vi "LeyboldPump_word.vi"() -> ()   [LabVIEW 2015]
panel:
  in  "PZD6 - Current intermediate circuit voltage 2":string="\u0000\u0000"
  in  "Reserved x2 2":string="\u0000\u0000"
  in  "PZD4 - Current Motor Current 2":string="\u0000\u0000"
  in  "PZD3 - Current Freq Converter Temp 2":string="\u0000\u0000"
  in  "PZD2 - Current Stator Freq 2":string="\u0000\u0000"
  in  "PZD1 - Status & Control 2":string="\u0000\u0000"
  in  "PWE (Parameter Value 4Bytes) 2":string="\u0000\u0000\u0000\u0000"
  in  "IND (Parameter Index) 2":string="\u0000"
  in  "Reserved 2":string="\u0000"
  in  "PKE - 2Bytes 2":string="\u0000\u0000"
  in  "ADR 2":string="\u0000"
  in  "LGE 2":string="\u0016"
  in  "STX 2":string="\u0002"
  out "Result String":string
  out "BCC - Checksum":string
  out "PZD6 - Current intermediate circuit voltage":string
  out "Reserved x2":string
  out "PZD4 - Current Motor Current":string
  out "PZD3 - Current Freq Converter Temp":string
  out "PZD2 - Current Stator Freq":string
  out "PZD1 - Status & Control":string
  out "PWE (Parameter Value 4Bytes)":string
  out "IND (Parameter Index)":string
  out "Reserved":string
  out "PKE - 2Bytes":string
  out "ADR":string
  out "LGE":string
  out "STX":string
  in  "Input String":string
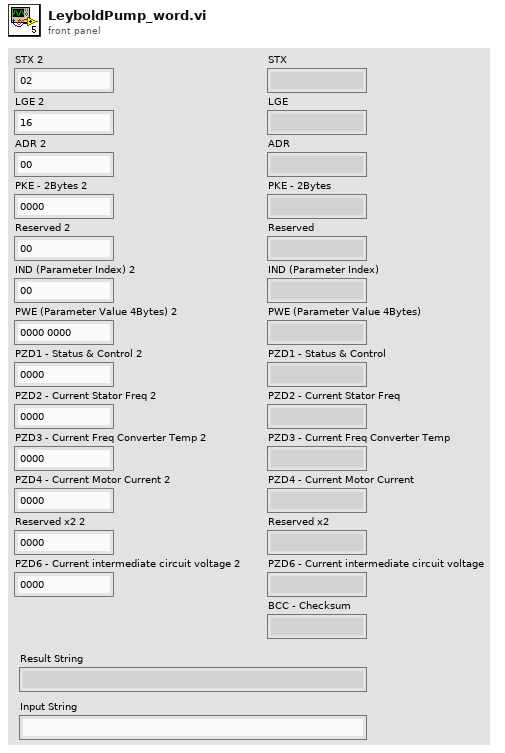
[diagram p1: front panel]
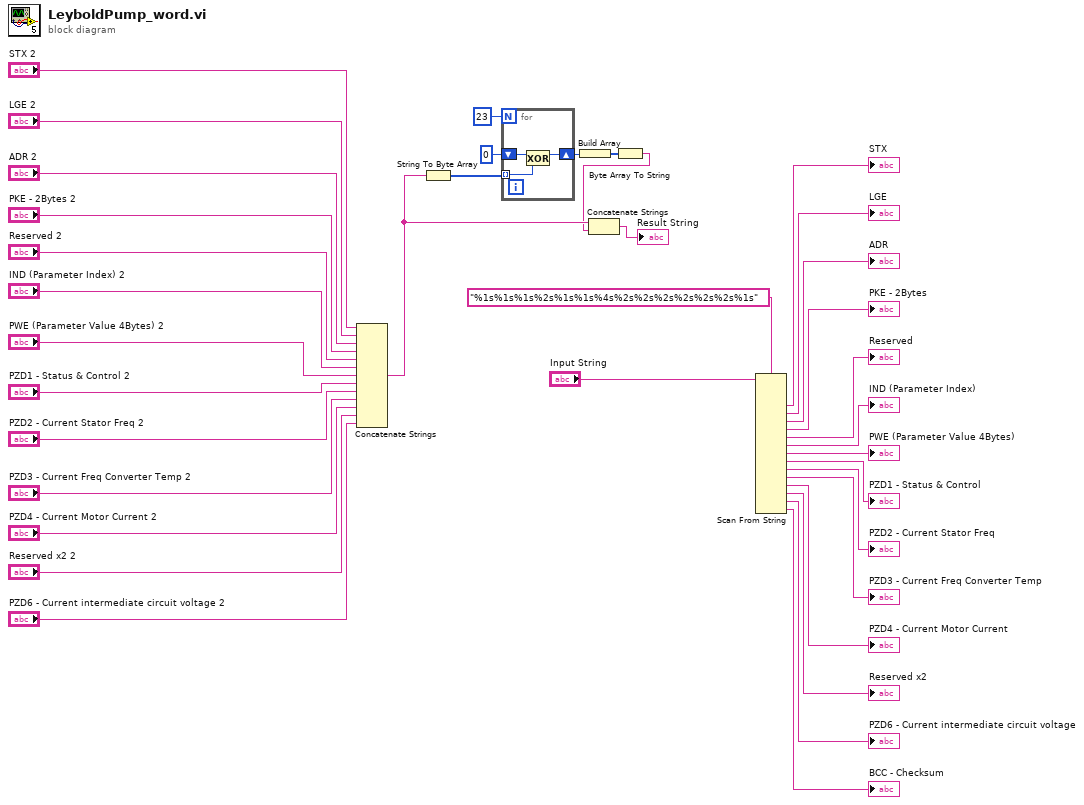
[diagram p0: block diagram]
diagram:
  n1 = Concatenate Strings("STX 2", "LGE 2", "ADR 2", "PKE - 2Bytes 2", "Reserved 2", "IND (Parameter Index) 2", "PWE (Parameter Value 4Bytes) 2", "PZD1 - Status & Control 2", "PZD2 - Current Stator Freq 2", "PZD3 - Current Freq Converter Temp 2", "PZD4 - Current Motor Current 2", "Reserved x2 2", "PZD6 - Current intermediate circuit voltage 2") -> (w4:string)
  n2 = String To Byte Array(string=w4) -> (unsigned byte array=w5:u8[])
  n3 = for {
    N: 23 -> [_]
    tunnel: w5 -> [w39] mode=indexing
    shift-right: [w38] -> w3
    shift-left: u8 0 -> [w40]
    n4 = Exclusive Or(1:w39, 2:w40) -> (0:w38:u8)
  }
  n5 = Build Array(w3) -> (w2:u8[])
  n6 = Byte Array To String(unsigned byte array=w2) -> (string=w1:string)
  n7 = Concatenate Strings(w4, w1) -> (→"Result String":string)
  n8 = Scan From String(format string="%1s%1s%1s%2s%1s%1s%4s%2s%2s%2s%2s%2s%2s%1s", input string="Input String") -> (output 1=→"STX":string, output 2=→"LGE":string, output 3=→"ADR":string, output 4=→"PKE - 2Bytes":string, output 5=→"Reserved":string, output 6=→"IND (Parameter Index)":string, output 7=→"PWE (Parameter Value 4Bytes)":string, output 8=→"PZD1 - Status & Control":string, output 9=→"PZD2 - Current Stator Freq":string, output 10=→"PZD3 - Current Freq Converter Temp":string, output 11=→"PZD4 - Current Motor Current":string, output 12=→"Reserved x2":string, output 13=→"PZD6 - Current intermediate circuit voltage":string, output 14=→"BCC - Checksum":string)  [unwired: 16 in, 3 out]
